vi "ImportComsolPotentials.vi"(0 "System":u16(ring) items=["Cusp", "Positron", "Musashi"]) -> (1 "# electrodes":i32=11, 2 "z (m)":dbl[](array[numeric])=[-0.54, -0.53878743, -0.53757487, -0.5363623, -0.53514974, -0.53393717, -0.53272461, -0.53151204, -0.53029948, -0.52908691, -0.52787435, -0.52666178, -0.52544922, -0.52423665, -0.52302409, -0.52181152, -0.52059896, -0.51938639, -0.51817382, -0.51696126, -0.51574869, -0.51453613, -0.51332356, -0.512111, -0.51089843, -0.50968587, -0.5084733, -0.50726074, -0.50604817, -0.50483561, -0.50362304, -0.50241048, -0.50119791, -0.49998535, -0.49877278, -0.49756022, -0.49634765, -0.49513508, -0.49392252, -0.49270995, -0.49149739, -0.49028482, -0.48907226, -0.48785969, -0.48664713, -0.48543456, -0.484222, -0.48300943, -0.48179687, -0.4805843, -0.47937174, -0.47815917, -0.47694661, -0.47573404, -0.47452147, -0.47330891, -0.47209634, -0.47088378, -0.46967121, -0.46845865, -0.46724608, -0.46603352, -0.46482095, -0.46360839, -0.46239582, -0.46118326, -0.45997069, -0.45875813, -0.45754556, -0.456333, -0.45512043, -0.45390786, -0.4526953, -0.45148273, -0.45027017, -0.4490576, -0.44784504, -0.44663247, -0.44541991, -0.44420734, -0.44299478, -0.44178221, -0.44056965, -0.43935708, -0.43814452, -0.43693195, -0.43571939, -0.43450682, -0.43329426, -0.43208169, -0.43086912, -0.42965656, -0.42844399, -0.42723143, -0.42601886, -0.4248063, -0.42359373, -0.42238117, -0.4211686, -0.41995604, -0.41874347, -0.41753091, -0.41631834, -0.41510578, -0.41389321, -0.41268065, -0.41146808, -0.41025551, -0.40904295, -0.40783038, -0.40661782, -0.40540525, -0.40419269, -0.40298012, -0.40176756, -0.40055499, -0.39934243, -0.39812986, -0.3969173, -0.39570473, -0.39449217, -0.3932796, -0.39206704, -0.39085447, -0.38964191, -0.38842934, -0.38721677, -0.38605446, -0.38489215, -0.38372984, -0.38256753, -0.38140522, -0.38024291, -0.3790806, -0.37791829, -0.37675598, -0.37574252, -0.37472906, -0.3737156, -0.37270214, -0.37168867, -0.37067521, -0.36966175, -0.36864829, -0.36763482, -0.36677864, -0.36592245, -0.36506626, -0.36421007, -0.36335388, -0.36249769, -0.3616415, -0.36078531, -0.35992912, -0.35909174, -0.35825437, -0.35741699, -0.35657961, -0.35574224, -0.35490486, -0.35406748, -0.35323011, -0.35239273, -0.35161386, -0.350835, -0.35005613, -0.34927726, -0.3484984, -0.34771953, -0.34694066, -0.3461618, -0.34538293, -0.34468681, -0.34399069, -0.34329457, -0.34259845, -0.34190233, -0.34120621, -0.34051008, -0.33981396, -0.33911784, -0.3384344, -0.33775095, -0.33706751, -0.33638406, -0.33570061, -0.33501717, -0.33433372, -0.33365028, -0.33296683, -0.33228338, -0.33159994, -0.33091649, -0.33023305, -0.3295496, -0.32886615, -0.32818271, -0.32749926, -0.32681582, -0.32613237, -0.32544893, -0.32476548, -0.32408203, -0.32339859, -0.32271514, -0.3220317, -0.32134825, -0.3206648, -0.31998136, -0.31929791, -0.31861447, -0.31793102, -0.31724757, -0.31656413, -0.31588068, -0.31519724, -0.31451379, -0.31383035, -0.3131469, -0.31246345, -0.31178001, -0.31109656, -0.31041312, -0.30972967, -0.30904622, -0.30836278, -0.30767933, -0.30699589, -0.30631244, -0.30562899, -0.30494555, -0.3042621, -0.30357866, -0.30289521, -0.30221177, -0.30152832, -0.30084487, -0.30016143, -0.29947798, -0.29879454, -0.29811109, -0.29742764, -0.2967442, -0.29606075, -0.29537731, -0.29469386, -0.29401041, -0.29332697, -0.29264352, -0.29196008, -0.29127663, -0.29059319, -0.28990974, -0.28922629, -0.28854285, -0.2878594, -0.28717596, -0.28649251, -0.28580906, -0.28512562, -0.28444217, -0.28375873, -0.28307528, -0.28239183, -0.28170839, -0.28102494, -0.2803415, -0.27965805, -0.27897461, -0.27829116, -0.27760771, -0.27692427, -0.27624082, -0.27555738, -0.27487393, -0.27419048, -0.27350704, -0.27282359, -0.27214015, -0.2714567, -0.27077325, -0.27008981, -0.26940636, -0.26872292, -0.26803947, -0.26735602, -0.26667258, -0.26598913, -0.26530569, -0.26462224, -0.2639388, -0.26325535, -0.2625719, -0.26188846, -0.26120501, -0.26052157, -0.25983812, -0.25915467, -0.25847123, -0.25778778, -0.25710434, -0.25642089, -0.25573744, -0.255054, -0.25437055, -0.25368711, -0.25300366, -0.25232022, -0.25163677, -0.25095332, -0.25026988, -0.24958643, -0.24890299, -0.24821954, -0.24753609, -0.24685265, -0.2461692, -0.24548576, -0.24480231, -0.24411886, -0.24343542, -0.24275197, -0.24206853, -0.24138508, -0.24070164, -0.24001819, -0.23933474, -0.2386513, -0.23796785, -0.23728441, -0.23660096, -0.23591751, -0.23523407, -0.23455062, -0.23386718, -0.23318373, -0.23250028, -0.23181684, -0.23113339, -0.23044995, -0.2297665, -0.22908306, -0.22839961, -0.22771616, -0.22703272, -0.22634927, -0.22566583, -0.22498238, -0.22429893, -0.22361549, -0.22293204, -0.2222486, -0.22156515, -0.2208817, -0.22019826, -0.21951481, -0.21883137, -0.21814792, -0.21746448, -0.21678103, -0.21609758, -0.21541414, -0.21473069, -0.21404725, -0.2133638, -0.21268035, -0.21199691, -0.21131346, -0.21063002, -0.20994657, -0.20926312, -0.20857968, -0.20789623, -0.20721279, -0.20652934, -0.2058459, -0.20516245, -0.204479, -0.20379556, -0.20311211, -0.20242867, -0.20174522, -0.20106177, -0.20037833, -0.19969488, -0.19901144, -0.19832799, -0.19764454, -0.1969611, -0.19627765, -0.19559421, -0.19491076, -0.19422732, -0.19354387, -0.19286042, -0.19217698, -0.19149353, -0.19081009, -0.19012664, -0.18944319, -0.18875975, -0.1880763, -0.18739286, -0.18670941, -0.18602596, -0.18534252, -0.18465907, -0.18397563, -0.18329218, -0.18260874, -0.18192529, -0.18124184, -0.1805584, -0.17987495, -0.17919151, -0.17850806, -0.17782461, -0.17714117, -0.17645772, -0.17577428, -0.17509083, -0.17440738, -0.17372394, -0.17304049, -0.17235705, -0.1716736, -0.17099016, -0.17030671, -0.16962326, -0.16893982, -0.16825637, -0.16757293, -0.16688948, -0.16620603, -0.16552259, -0.16483914, -0.1641557, -0.16347225, -0.1627888, -0.16210536, -0.16142191, -0.16073847, -0.16005524, -0.15937201, -0.15868879, -0.15800556, -0.15732233, -0.15663911, -0.15595588, -0.15527265, -0.15458943, -0.15394982, -0.15331021, -0.1526706, -0.15203099, -0.15139139, -0.15075178, -0.15011217, -0.14947256, -0.14883295, -0.14826376, -0.14769457, -0.14712537, -0.14655618, -0.14598698, -0.14541779, -0.1448486, -0.1442794, -0.14371021, -0.1432267, -0.14274319, -0.14225968, -0.14177617, -0.14129266, -0.14080916, -0.14032565, -0.13984214, -0.13935863, -0.13896152, -0.13856441, -0.1381673, -0.13777018, -0.13737307, -0.13697596, -0.13657885, -0.13618174, -0.13578463, -0.13545856, -0.1351325, -0.13480644, -0.13448037, -0.13415431, -0.13382825, -0.13350219, -0.13317612, -0.13285006, -0.13257918, -0.13230829, -0.13203741, -0.13176653, -0.13149564, -0.13122476, -0.13095388, -0.130683, -0.13041211, -0.13018235, -0.12995259, -0.12972282, -0.12949306, -0.1292633, -0.12903354, -0.12880377, -0.12857401, -0.12834425, -0.12814936, -0.12795448, -0.12775959, -0.12756471, -0.12736983, -0.12717494, -0.12698006, -0.12678517, -0.12659029, -0.12642499, -0.12625969, -0.12609438, -0.12592908, -0.12576378, -0.12559848, -0.12543318, -0.12526788, -0.12510258, -0.12496237, -0.12482216, -0.12468196, -0.12454175, -0.12440154, -0.12426133, -0.12412112, -0.12398091, -0.12384071, -0.12372178, -0.12360286, -0.12348393, -0.12336501, -0.12324609, -0.12312716, -0.12300824, -0.12288931, -0.12277039, -0.12266939, -0.1225684, -0.12246741, -0.12236641, -0.12226542, -0.12216442, -0.12206343, -0.12196244, -0.12186144, -0.12176664, -0.12167184, -0.12157704, -0.12148224, -0.12138744, -0.12129264, -0.12119784, -0.12110304, -0.12100824, -0.12091344, -0.12081864, -0.12072384, -0.12062904, -0.12053424, -0.12043943, -0.12034463, -0.12024983, -0.12015503, -0.12006023, -0.11996543, -0.11987063, -0.11977583, -0.11968103, -0.11958623, -0.11949143, -0.11939663, -0.11930183, -0.11920703, -0.11911223, -0.11901743, -0.11892263, -0.11882782, -0.11873302, -0.11863822, -0.11854342, -0.11844862, -0.11835382, -0.11825902, -0.11816422, -0.11806942, -0.11797462, -0.11787982, -0.11778502, -0.11769022, -0.11759542, -0.11750062, -0.11740582, -0.11731102, -0.11721622, -0.11712141, -0.11702661, -0.11693181, -0.11683701, -0.11674221, -0.11664741, -0.11655261, -0.11645781, -0.11636301, -0.11626821, -0.11617341, -0.11607861, -0.11598381, -0.11588901, -0.11579421, -0.11569941, -0.11560461, -0.11550981, -0.115415, -0.1153202, -0.1152254, -0.1151306, -0.1150358, -0.114941, -0.1148462, -0.1147514, -0.1146566, -0.1145618, -0.114467, -0.1143722, -0.1142774, -0.1141826, -0.1140878, -0.113993, -0.1138982, -0.1138034, -0.11370859, -0.11361379, -0.11351899, -0.11342419, -0.11332939, -0.11323459, -0.11313979, -0.11304499, -0.11295019, -0.11285539, -0.11276059, -0.11266579, -0.11257099, -0.11247619, -0.11238139, -0.11228659, -0.11219179, -0.11209699, -0.11200218, -0.11190738, -0.11181258, -0.11171778, -0.11162298, -0.11152746, -0.11143195, -0.11133643, -0.11124091, -0.11114539, -0.11104988, -0.11095436, -0.11085884, -0.11076332, -0.11065501, -0.1105467, -0.11043839, -0.11033008, -0.11022177, -0.11011345, -0.11000514, -0.10989683, -0.10978852, -0.10966082, -0.10953313, -0.10940543, -0.10927774, -0.10915004, -0.10902235, -0.10889465, -0.10876695, -0.10863926, -0.10848871, -0.10833816, -0.10818761, -0.10803706, -0.10788651, -0.10773596, -0.10758542, -0.10743487, -0.10728432, -0.10710682, -0.10692933, -0.10675184, -0.10657435, -0.10639685, -0.10621936, -0.10604187, -0.10586438, -0.10568688, -0.10547762, -0.10526837, -0.10505911, -0.10484985, -0.10464059, -0.10443133, -0.10422207, -0.10401282, -0.10380356, -0.10355685, -0.10331014, -0.10306343, -0.10281672, -0.10257001, -0.1023233, -0.1020766, -0.10182989, -0.10158318, -0.10129088, -0.10099859, -0.10070629, -0.100414, -0.1001217, -0.09982941, -0.099537115, -0.09924482, -0.098952525, -0.098597407, -0.098242289, -0.097887171, -0.097532053, -0.097176935, -0.096821817, -0.096466699, -0.096111581, -0.095756463, -0.095324084, -0.094891705, -0.094459327, -0.094026948, -0.093594569, -0.09316219, -0.092729811, -0.092297432, -0.091865053, -0.091337838, -0.090810622, -0.090283406, -0.089756191, -0.089228975, -0.088701759, -0.088174543, -0.087647328, -0.087120112, -0.086476765, -0.085833418, -0.085190071, -0.084546724, -0.083903377, -0.08326003, -0.082616683, -0.081973336, -0.081329989, -0.080545643, -0.079761297, -0.07897695, -0.078192604, -0.077408258, -0.076623912, -0.075839566, -0.075055219, -0.074270873, -0.073314982, -0.072359091, -0.071403199, -0.070447308, -0.069491417, -0.068535526, -0.067579634, -0.066623743, -0.065667852, -0.064535704, -0.063403557, -0.06227141, -0.061139262, -0.060007115, -0.058874967, -0.05774282, -0.056610673, -0.055478525, -0.05426596, -0.053053395, -0.051840829, -0.050628264, -0.049415699, -0.048203134, -0.046990568, -0.045778003, -0.044565438, -0.043352872, -0.042140307, -0.040927742, -0.039715177, -0.038502611, -0.037290046, -0.036077481, -0.034864915, -0.03365235, -0.032439785, -0.03122722, -0.030014654, -0.028802089, -0.027589524, -0.026376958, -0.025164393, -0.023951828, -0.022739263, -0.021526697, -0.020314132, -0.019101567, -0.017889001, -0.016676436, -0.015463871, -0.014251306, -0.01303874, -0.011826175, -0.01061361, -0.0094010445, -0.0081884792, -0.006975914, -0.0057633487, -0.0045507834, -0.0033382181, -0.0021256528, -0.00091308754, 0.00029947774, 0.001512043, 0.0027246083, 0.0039371736, 0.0051497389, 0.0063623042, 0.0075748694, 0.0087874347], 3 "V(z)":dbl[][](array[numeric]))   [LabVIEW 2018]
panel:
  in  "ComsolPotsFilename":string="ComsolPots.csv"
  out "all rows":dbl[][](array[numeric]) format="%_5e"
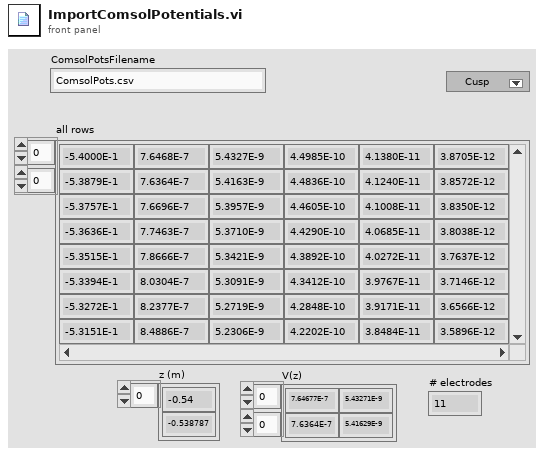
[diagram p1: front panel]
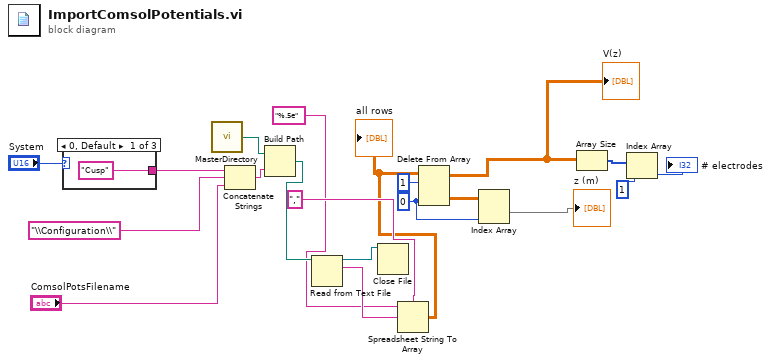
[diagram p0: block diagram]
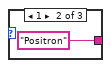
[diagram p2: hidden frame]
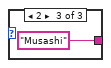
[diagram p3: hidden frame]
diagram:
  w18 = 0 ("disabled index (col)")
  n1 = case shown="0, Default" "System" {
    tunnel: ["Cusp" ("string") "Positron" ("string") "Musashi" ("string")] -> w15
    frame 0, Default {
    }
    frame 1 {
    }
    frame 2 {
    }
  }
  n2 = call "MasterDirectory.vi"() -> ("Master Directory"=w13:path)
  n3 = Concatenate Strings(w15, "\\Configuration\\", "ComsolPotsFilename") -> (w12:string)
  n4 = Build Path(base path=w13, name or relative path=w12) -> (appended path=w6:path)
  n5 = Read from Text File(file (use dialog)=w6) -> (refnum out=w5:refnum<file>, text=w4:string)  [unwired: 3 in, 2 out]
  n6 = Close File(refnum=w5) -> ()  [unwired: 1 in, 2 out]
  n7 = Spreadsheet String To Array(delimiter (Tab)="," ("delimiter (\\t)"), format string="%.5e" ("format (%.3f)"), spreadsheet string=w4) -> (array=w1:dbl[][])  [unwired: 1 in]
  "all rows" <- w1
  n8 = Delete From Array(array=w1, length=1, index (col)=w18) -> (deleted portion=w19:dbl[][], array with subset deleted=w8:dbl[][])  [unwired: 1 in]
  "V(z)" <- w8
  n9 = Index Array(array=w19, index (col)=w18) -> (element=→"z (m)":dbl[])  [unwired: 1 in]
  n10 = Array Size(array=w8) -> (size(s)=w17:i32[])
  n11 = Index Array(array=w17, index=1) -> (element=→"# electrodes":i32)
